vi "Configure Channel (Voltage)_TJV.vi"(0 "VISA resource name":refnum<visa-resource-name>, 1 "Current Range:\n0=1uA\n1=10uA\n2=100uA\n3=1mA\n4=10mA\n5=120mA":i32=5, 2 "Channel (1: Channel 1)":u16(ring)=1 items=["Channel 1"=1, "Channel 2"=2, "Channel 3"=3], 5 "Stabilization Voltage(V)":dbl=1.0, 7 "Probe Voltage(V)":dbl=1.0, 11 "error in (no error)":errorcluster, 12 "Voltage Range (0: 2 Volts)":u16(ring) items=["2 Volts", "20 Volts"], 13 "Time Interval (ms)":i32, 14 "Number of points (max 4096)":i32) -> (4 "VISA resource name out":refnum<visa-resource-name>, 6 "Actual Current Level (A)":dbl[](array[numeric]) format="%.2g", 15 "error out":errorcluster)   [LabVIEW 2018, in "Agilent U2722.lvlib"]
doc: "Configures the channel to output in source voltage mode."
uses:
  Agilent U2722.lvlib
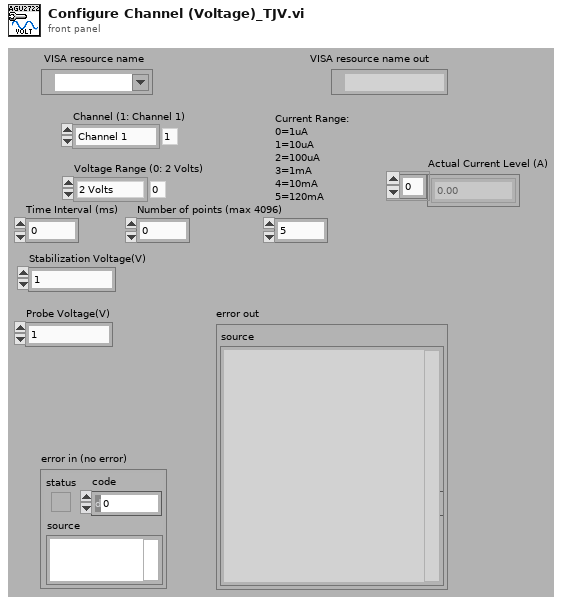
[diagram p1: front panel]
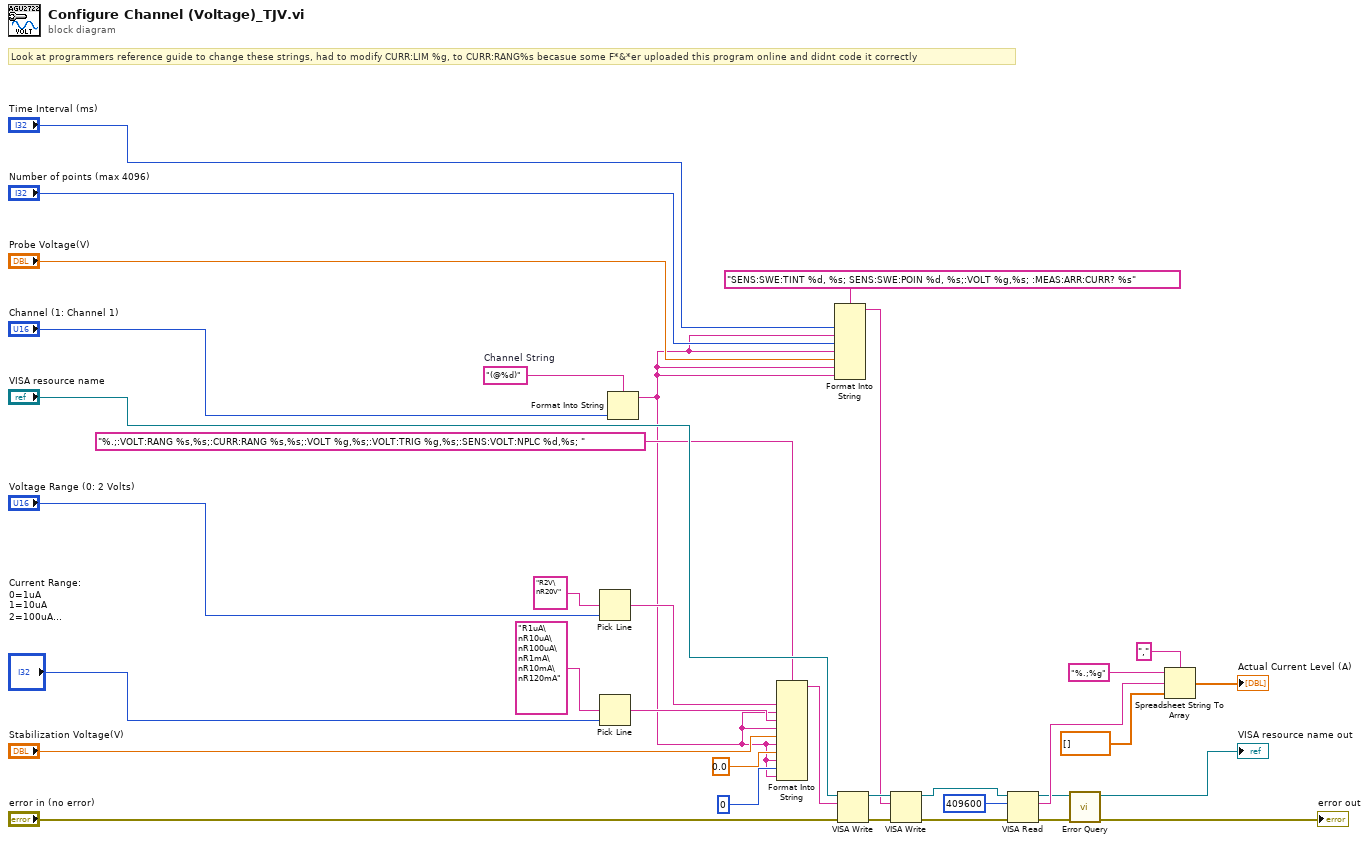
[diagram p0: block diagram]
diagram:
  w30 = "(@%d)"  # Channel String
  # "Look at programmers reference guide to change these strings, had to modify CURR:LIM %g, to CURR:RANG%s becasue some F*&*er uploaded this program online and didnt code it correctly"
  n1 = Pick Line(multi-line string="R2V\nR20V", line index="Voltage Range (0: 2 Volts)") -> (output string=w25:string)  [unwired: 1 in]
  n2 = Pick Line(multi-line string="R1uA\nR10uA\nR100uA\nR1mA\nR10mA\nR120mA", line index="Current Range:\n0=1uA\n1=10uA\n2=100uA\n3=1mA\n4=10mA\n5=120mA") -> (output string=w23:string)  [unwired: 1 in]
  n3 = Format Into String(format string=w30, "Channel (1: Channel 1)") -> (resulting string=w2:string)  [unwired: 2 in, 1 out]
  n4 = Format Into String(format string="%.;:VOLT:RANG %s,%s;:CURR:RANG %s,%s;:VOLT %g,%s;:VOLT:TRIG %g,%s;:SENS:VOLT:NPLC %d,%s; ", w25, w2, w23, w2, "Stabilization Voltage(V)", w2, 0.0 ("input 7"), w2, 0 ("Power Line Cycles (0)"), w2) -> (resulting string=w28:string)  [unwired: 2 in, 1 out]
  n5 = Format Into String(format string="SENS:SWE:TINT %d, %s; SENS:SWE:POIN %d, %s;:VOLT %g,%s; :MEAS:ARR:CURR? %s", "Time Interval (ms)", w2, "Number of points (max 4096)", w2, "Probe Voltage(V)", w2, w2) -> (resulting string=w1:string)  [unwired: 2 in, 1 out]
  n6 = VISA Write(VISA resource name="VISA resource name", write buffer=w28, error in (no error)="error in (no error)") -> (VISA resource name out=w9:refnum<visa-resource-name>, error out=w8:errorcluster)  [unwired: 1 out]
  n7 = VISA Write(VISA resource name=w9, write buffer=w1, error in (no error)=w8) -> (VISA resource name out=w6:refnum<visa-resource-name>, error out=w7:errorcluster)  [unwired: 1 out]
  n8 = VISA Read(VISA resource name=w6, byte count=u32 409600, error in (no error)=w7) -> (VISA resource name out=w13:refnum<visa-resource-name>, read buffer=w16:string, error out=w14:errorcluster)  [unwired: 1 out]
  n9 = call "Error Query.vi"("error in (no error)"=w14, "VISA resource name"=w13) -> ("error out"=→"error out":errorcluster, "VISA resource name out"=→"VISA resource name out":refnum<visa-resource-name>)  [unwired: 6 in, 2 out]
  n10 = Spreadsheet String To Array(delimiter (Tab)=",", format string="%.;%g", spreadsheet string=w16, array type (2D Dbl)=dbl[] []) -> (array=→"Actual Current Level (A)":dbl[])
